vi "Last Ack.vi"(10 "Actor":refnum<class "Actor.lvclass">, 11 "jettl in":refnum<class "jettl.lvclass">) -> (3 "jettl out":refnum<class "jettl.lvclass">)   [LabVIEW 2021, in "jettl.lvlib" / "jettl.lvclass"]
uses:
  jettl.lvclass
  Actor/Actor.lvclass
  jettl.lvclass/jettl.ctl
  jettl.lvlib
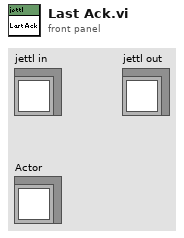
[diagram p1: front panel]
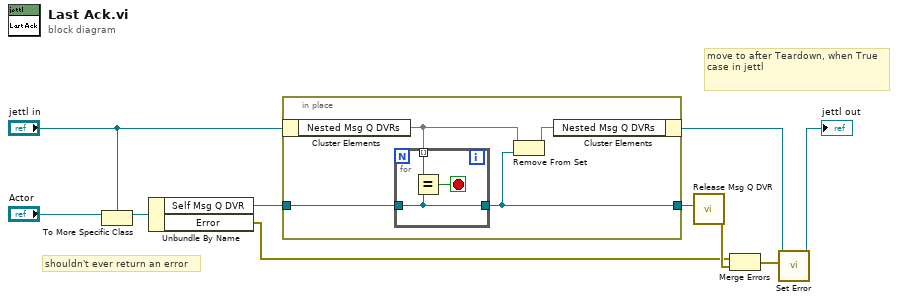
[diagram p0: block diagram]
diagram:
  # "move to after Teardown, when True case in jettl"
  # "shouldn't ever return an error"
  n1 = To More Specific Class(target class="jettl in", reference="Actor") -> (specific class reference=w10:refnum<class "jettl.lvclass">)  [unwired: 1 in, 1 out]
  n2 = Unbundle By Name(w10) -> ("Self Msg Q DVR"=w8:refnum<data-value>, "Error"=w5:errorcluster)
  n3 = in-place {
    in-place-border: w8 -> [w12]
    in-place-border: [w11] -> w7
    n4 = in-place-cluster #1("jettl in") -> ("Nested Msg Q DVRs"=w14:set{refnum<data-value>})
    n5 = for {
      tunnel: w12 -> [w15]
      tunnel: w14 -> [w16] mode=indexing
      tunnel: [w15] -> w11
      stop <- w17 stop-if-true
      n6 = Equal?(x=w16, y=w15) -> (x = y?=w17:bool)
    }
    n7 = Remove From Set(10:w11, 11:w14) -> (3:w13:set{refnum<data-value>})  [unwired: 1 out]
    n8 = in-place-cluster #1("Nested Msg Q DVRs"=w13) -> (w4:refnum<class "jettl.lvclass">)
  }
  n9 = call "Release Msg Q DVR.vi"("Msg Q DVR"=w7) -> ("error out"=w6:errorcluster)  [unwired: 10 in]
  n10 = Merge Errors(w5, w6) -> (w2:errorcluster)
  n11 = call-dynamic "Set Error.vi"("Error"=w2, "jettl in"=w4) -> ("jettl out"=→"jettl out":refnum<class "jettl.lvclass">)  [unwired: 9 in]
